vi "Find Min (SubVI).vi"(10 "Data 2":u8, 11 "Data 1":u8) -> (3 "Min":u8)   [LabVIEW 2015]
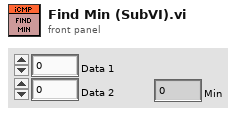
[diagram p1: front panel]
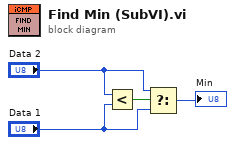
[diagram p0: block diagram]
diagram:
  n1 = Less?(x="Data 2", y="Data 1") -> (x < y?=w2:bool)
  n2 = Select(t="Data 2", s=w2, f="Data 1") -> (s? t:f=→"Min":u8)
